vi "Read Loop.vi"(11 "Telemetry Server in":refnum<class "Telemetry Server.lvclass">) -> ()   [LabVIEW 2020, in "VolatusTelemetry.lvlib" / "Telemetry Server.lvclass"]
uses:
  Telemetry Server.lvclass
  Telemetry Server.lvclass/Telemetry Server.ctl
  messages/UdpPayload/UdpPayload.lvlib
  IPv4 Endpoint.ctl
  Volatus/MessageQ/MessageQ.lvclass
  Volatus/Module/Module.lvclass
  C:/dev/lv20CE/relink/lv-volatus/Volatus/Module/Module.lvclass
  C:/dev/lv20CE/relink/lv-volatus/VolatusTelemetry/Telemetry Server/Telemetry Server.lvclass
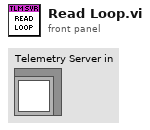
[diagram p1: front panel]
types:
  T1 = typedef "VolatusTelemetry.lvlib/Telemetry Server.lvclass/IPv4 Endpoint.ctl" = cluster{"Address":u32, "Port":u16}
  T2 = typedef "UdpPayload.lvlib/Data.ctl" = cluster{"source_id":u32, "sequence":u32, "timestamp":i64, "type":string, "payload":u8[]}
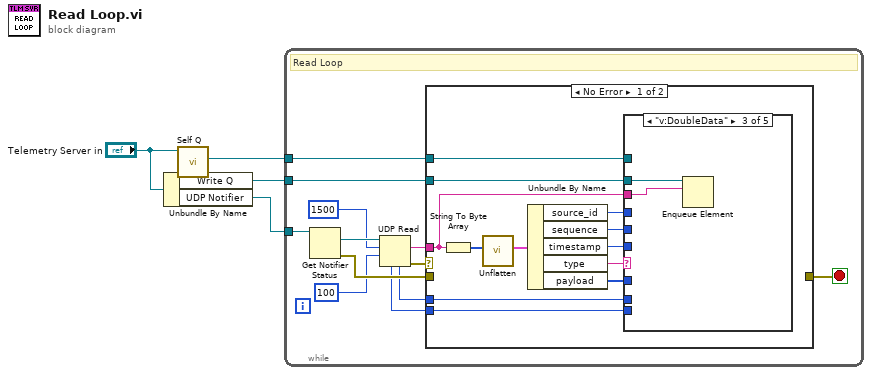
[diagram p0: block diagram]
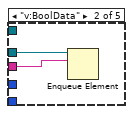
[diagram p3: hidden frame]
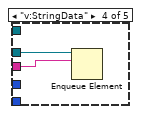
[diagram p4: hidden frame]
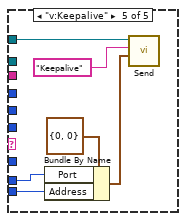
[diagram p5: hidden frame]
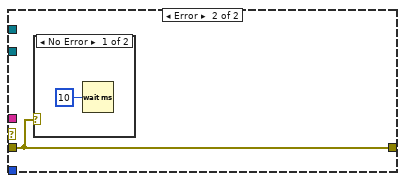
[diagram p6: hidden frame]
diagram:
  n1 = Unbundle By Name("Telemetry Server in") -> ("Write Q"=w3:refnum<queue>, "UDP Notifier"=w1:refnum<notifier>)
  n2 = call "Self Q.vi"("Module in"="Telemetry Server in") -> ("Self Q"=w4:refnum<class "MessageQ.lvclass">)  [unwired: 9 in, 1 out]
  n3 = while {
    tunnel: w4 -> [w7]
    tunnel: w3 -> [w6]
    tunnel: w1 -> [w5]
    stop <- w8 stop-if-true
    # "Read Loop"
    n4 = Get Notifier Status(notifier=w5) -> (current notification=w15:refnum<k16>, error out=w16:errorcluster)  [unwired: 1 in, 3 out]
    n5 = UDP Read(connection ID=w15, max size (548)=1500, timeout ms (25000)=100) -> (data out=w12:string, error out=w13:errorcluster, 4:w9:u16, 6:w10:u32)  [unwired: 1 in, 1 out]
    n6 = case shown="No Error" w13 {
      tunnel: w12 -> [w19 _]
      tunnel: w10 -> [w20 _]
      tunnel: w9 -> [w21 _]
      tunnel: w16 -> [_ w41]
      tunnel: [_ w41] -> w8
      tunnel: w7 -> [w18 _]
      tunnel: w6 -> [w17 _]
      frame No Error {
        n7 = String To Byte Array(string=w19) -> (unsigned byte array=w28:u8[])
        n8 = call "Unflatten.vi"("Buffer"=w28) -> ("Data"=w27:T2)  [unwired: 9 in, 1 out]
        n9 = Unbundle By Name(w27) -> ("source_id"=w22:u32, "sequence"=w23:u32, "timestamp"=w24:i64, "type"=w26:string, "payload"=w25:u8[])
        n10 = case shown="\"v:DoubleData\"" w26 {
          tunnel: w25 -> [_ _ _ _ _]
          tunnel: w24 -> [_ _ _ _ _]
          tunnel: w23 -> [_ _ _ _ _]
          tunnel: w22 -> [_ _ _ _ _]
          tunnel: w21 -> [_ _ _ _ w39]
          tunnel: w20 -> [_ _ _ _ w38]
          tunnel: w19 -> [_ w30 w32 w34 _]
          tunnel: w18 -> [_ _ _ _ w35]
          tunnel: w17 -> [_ w29 w31 w33 _]
          frame Default {
          }
          frame "v:BoolData" {
            n11 = Enqueue Element(queue=w29, element=w30) -> ()  [unwired: 2 in, 3 out]
          }
          frame "v:DoubleData" {
            n12 = Enqueue Element(queue=w31, element=w32) -> ()  [unwired: 2 in, 3 out]
          }
          frame "v:StringData" {
            n13 = Enqueue Element(queue=w33, element=w34) -> ()  [unwired: 2 in, 3 out]
          }
          frame "v:Keepalive" {
            n14 = Bundle By Name(cluster=T1 {"Address"=0, "Port"=0} ("IPv4 Endpoint"), "Port"=w39, "Address"=w38) -> (w37:T1)
            n15 = call "Send.vi"("Data"=w37, "ID"="Keepalive", "MessageQ in"=w35) -> ()  [unwired: 7 in, 2 out]
          }
        }
      }
      frame Error {
        n16 = case shown="No Error" w41 {
          frame No Error {
            n17 = Wait (ms)(milliseconds to wait=u32 10) -> ()  [unwired: 1 out]
          }
          frame Error {
          }
        }
      }
    }
  }
